vi "DoubleClick Callback.vi"(4 "onDoubleClick":refnum<user-event>, 5 "Event Data":cluster{"sender":refnum<k24>, "e":refnum<k24>}, 6 "Control Ref":refnum<k24>, 7 "Event Common Data":T1) -> ()   [LabVIEW 2024, in "SourceGrid.lvlib" / "Custom Events.lvclass"]
uses:
  Custom Events.lvclass
  D:/git/Sourcegrid-LabVIEW/dll/SourceGrid.dll
  dll/SourceGrid.dll
  Cells/Cell Context/Cell Context.lvclass
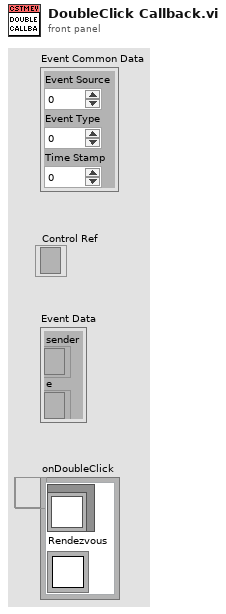
[diagram p1: front panel]
types:
  T1 = cluster{"Event Source":i32, "Event Type":u32, "Time Stamp":u32}
  T2 = typedef "Rendezvous RefNum" = refnum<k1>
  T3 = cluster{"Cell Context":refnum<class "Cell Context.lvclass">, "Rendezvous":T2}
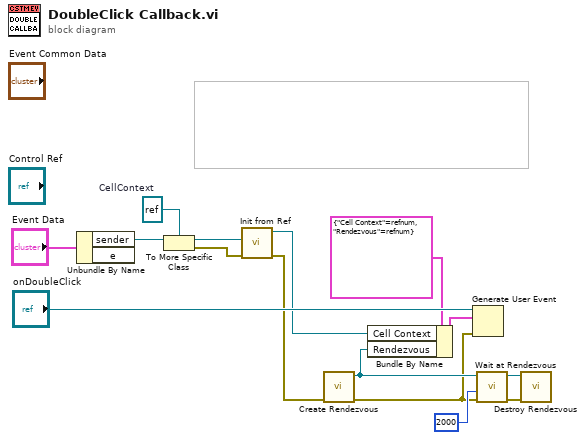
[diagram p0: block diagram]
diagram:
  w10 = refnum<k24> refnum  # CellContext
  n1 = Unbundle By Name("Event Data") -> ("sender"=w14:refnum<k24>)  [unwired: 1 out]
  n2 = To More Specific Class(target class=w10, reference=w14) -> (specific class reference=w11:refnum<k24>, error out=w13:errorcluster)  [unwired: 1 in]
  n3 = call "Init from Ref.vi"("error in"=w13, "CellContext .NET"=w11) -> ("error out"=w9:errorcluster, "Cell Context out"=w4:refnum<class "Cell Context.lvclass">)  [unwired: 8 in]
  n4 = call <vilib>:"Create Rendezvous.vi"("error in (no error)"=w9) -> ("error out"=w1:errorcluster, "rendezvous"=w5:T2)  [unwired: 4 in, 1 out]
  n5 = Bundle By Name(cluster=T3 {"Cell Context"=refnum, "Rendezvous"=refnum} ("onDoubleClick"), "Cell Context"=w4, "Rendezvous"=w5) -> (w6:T3)
  n6 = Generate User Event(user event="onDoubleClick", event data cluster=w6, error in=w1) -> ()  [unwired: 1 in, 2 out]
  n7 = call <vilib>:"Wait at Rendezvous.vi"("error in (no error)"=w1, "ms timeout (-1)"=2000, "rendezvous"=w5) -> ("error out"=w3:errorcluster, "rendezvous out"=w2:T2)  [unwired: 2 in, 1 out]
  n8 = call <vilib>:"Destroy Rendezvous.vi"("error in (no error)"=w3, "rendezvous"=w2) -> ()  [unwired: 4 in, 2 out]
